vi "createDataEvent.vi"(8 "error in (no error)":errorcluster, 9 "Callback VI Ref":refnum<vi>, 10 "Event Callback in":refnum<k27>, 11 "SM1000-control in":T1) -> (0 "error out":errorcluster, 2 "Event Callback":refnum<k27>, 3 "SM1000-control out":T1)   [LabVIEW 2013, in "SLMControl.lvlib" / "SM1000.lvclass"]
doc: "Registers for application and exception events returned from the EC device session.\nThe method 'handleConnectEvent' is called when the event is detected."
uses:
  SM1000.lvclass
  Object-reference.ctl
  SM1000.lvclass/SM1000.ctl
  Custom-errors.ctl
  C:/Users/vangeste/Desktop/2015-06-02 - SLM - MAIF/HC-HardwareCharacterization/Sources/SM1000/LECSession.dll
  HC-HardwareCharacterization/Sources/SM1000/LECSession.dll
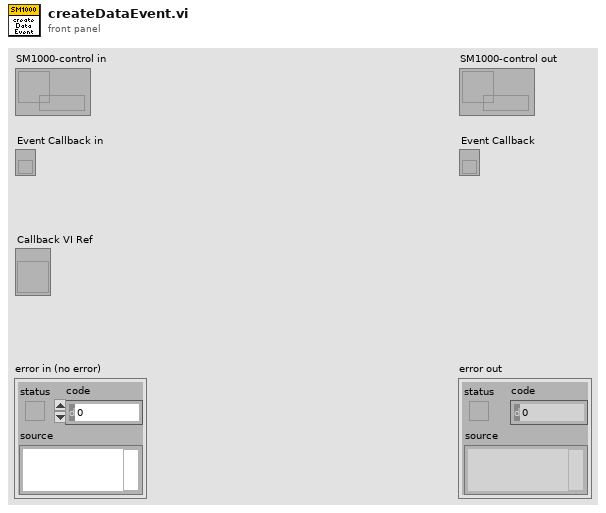
[diagram p1: front panel]
types:
  T1 = typedef "SLMControl.lvlib/SM1000.lvclass/Object-reference.ctl" = refnum<data-value>
  T2 = typedef "SLMControl.lvlib/SM1000.lvclass/Custom-errors.ctl" = enum16{"No error", "Not implemented", "Command not recognized", "Invalid input", "No connection", "Timeout", "Resource not loaded"}
  T3 = cluster{"puiPayloadHigh":u32, "puiPayloadLow":u32, "pstrData":string}
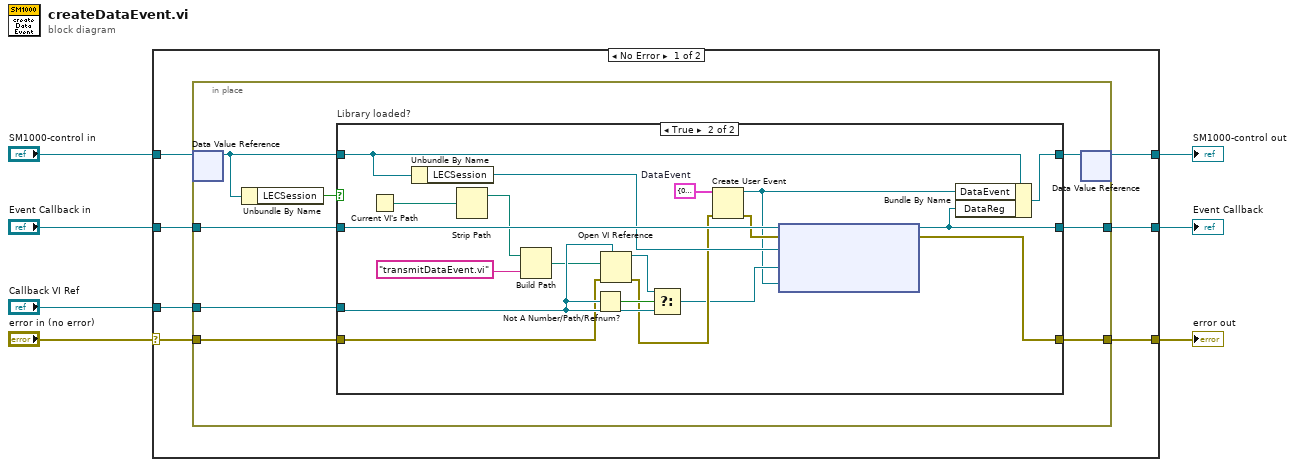
[diagram p0: block diagram]
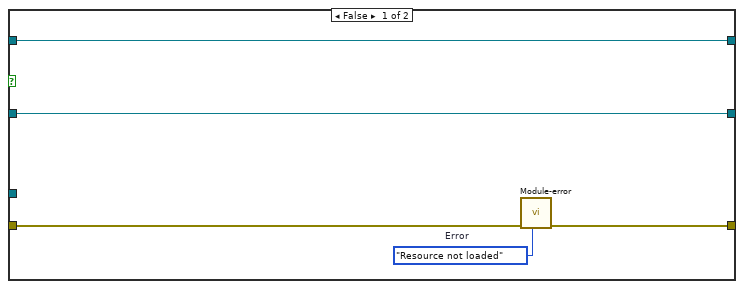
[diagram p2: hidden frame]
diagram:
  n1 = case shown="No Error" "error in (no error)" {
    selector: "error in (no error)" -> [w13 w49]
    tunnel: [w12 w49] -> w6
    tunnel: [w14 w48] -> w4
    tunnel: "SM1000-control in" -> [w8 w48]
    tunnel: "Event Callback in" -> [w11 w47]
    tunnel: "Callback VI Ref" -> [w10 _]
    tunnel: [w9 w47] -> w2
    frame No Error {
      n2 = in-place {
        in-place-border: w13 -> [w22]
        in-place-border: [w19] -> w12
        in-place-border: w11 -> [w17]
        in-place-border: w10 -> [w15]
        in-place-border: [w16] -> w9
        n3 = in-place-dvr #1(w8) -> (w20:refnum<class "SM1000.lvclass">)  [unwired: 1 out]
        n4 = Unbundle By Name(w20) -> ("LECSession"=w21:bool)
        n5 = case "Library loaded?" shown="True" w21 {
          tunnel: w22 -> [w27 w39]
          tunnel: w20 -> [w25 w46]
          tunnel: [w26 w32] -> w19
          tunnel: [w25 w35] -> w18
          tunnel: w17 -> [w24 w45]
          tunnel: w15 -> [_ w42]
          tunnel: [w24 w28] -> w16
          frame False {
            w23 = Custom-errors."Resource not loaded"  # Error
            n6 = call "Module-error.vi"("Error"=w23, "error in (no error)"=w27) -> ("error out"=w26:errorcluster)  [unwired: 9 in]
          }
          frame True {
            w31 = T3 {"puiPayloadHigh"=0, "puiPayloadLow"=0, "pstrData"=""}  # DataEvent
            n7 = Current VI's Path() -> (path=w37:path)
            n8 = Unbundle By Name(w46) -> ("LECSession"=w44:refnum<k24>)
            n9 = Strip Path(path=w37) -> (stripped path=w36:path)  [unwired: 1 out]
            n10 = Build Path(base path=w36, name or relative path="transmitDataEvent.vi") -> (appended path=w40:path)
            n11 = Not A Number/Path/Refnum?(number/path/refnum=w42) -> (NaN/Path/Refnum?=w43:bool)
            n12 = Open VI Reference(type specifier VI Refnum (for type only)=w42, vi path=w40, error in (no error)=w39) -> (vi reference=w38:refnum<vi>, error out=w34:errorcluster)  [unwired: 3 in]
            n13 = Select(t=w38, s=w43, f=w42) -> (s? t:f=w30:refnum<vi>)
            n14 = Create User Event(user event datatype=w31, error in=w34) -> (user event=w29:refnum<user-event>, error out=w33:errorcluster)
            n15 = node(w45, w33, w44, w30, w29) -> (w28:refnum<k27>, w32:errorcluster)
            n16 = Bundle By Name(cluster=w46, "DataEvent"=w29, "DataReg"=w28) -> (w35:refnum<class "SM1000.lvclass">)
          }
        }
        n17 = in-place-dvr #1(w18) -> (w14:T1)  [unwired: 1 out]
      }
    }
    frame Error {
    }
  }
  "error out" <- w6
  "SM1000-control out" <- w4
  "Event Callback" <- w2
